vi "arduino_LM35.vi"() -> ()   [LabVIEW 2018]
uses:
  <vilib>/MakerHub/LINX/Public/Peripherals/Analog/Analog Read 1 Chan.vi
  <vilib>/MakerHub/LINX/Public/Peripherals/Analog/Analog Read N Chans.vi
  <vilib>/MakerHub/LINX/Private/Local IO/LinxAnalogRead.vi
  <vilib>/MakerHub/LINX/Public/Utilities/Check Channel.vi
  <vilib>/MakerHub/LINX/Private/Utilties/Generate Error.vi
  <vilib>/MakerHub/LINX/LMH-LINX.lvlib
panel:
  out "Sıcaklık":dbl
  in  "stop":bool
  out "Sıcaklık Grafiği":dbl(graph)
  out "Sıcaklık":dbl(slide) scale=0.0..100.0
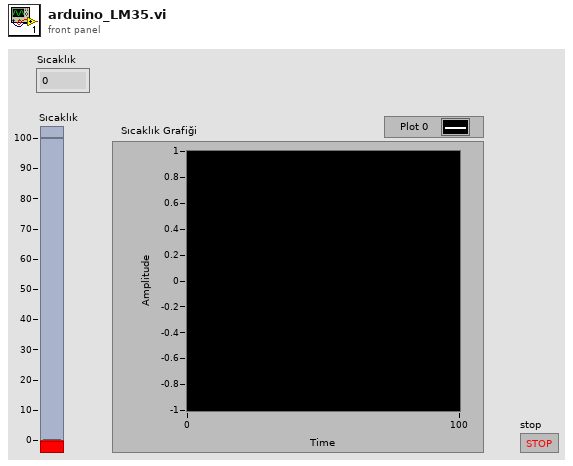
[diagram p1: front panel]
types:
  T1 = typedef "LMH-LINX.lvlib/LINX Ref.ctl" = cluster{"IO":T2, "Interface":T3, "LINX Device Config":T4}
  T2 = typedef "LMH-LINX.lvlib/Platform.ctl" = enum16{"Remote", "Local"}
  T3 = typedef "LMH-LINX.lvlib/Interface.ctl" = enum16{"Serial", "TCP"}
  T4 = typedef "LMH-LINX.lvlib/Device.lvlib/LINX Device Config.ctl" = cluster{"Interface":T3, "COM Port":refnum<visa-resource-name>, "TCP Configuration":T5, "Device Family":u8, "Device ID":u8, "Device Name":string, "TCP Ref":refnum<k5>, "Channels":T6}
  T5 = typedef "LMH-LINX.lvlib/Device.lvlib/TCP Config.ctl" = cluster{"IP Address":string, "Port":u16}
  T6 = typedef "LMH-LINX.lvlib/Channels.ctl" = cluster{"DI":u8[], "DO":u8[], "AI":u8[], "AO":u8[], "PWM":u8[], "QE":u8[], "UART":u8[], "I2C 2":u8[], "SPI":u8[], "CAN":u8[], "Servo":u8[], "AI Ref (V)":dbl, "AI Resolution (Bits)":u8, "AO Ref (V)":dbl, "AO Resolution (Bits)":u8}
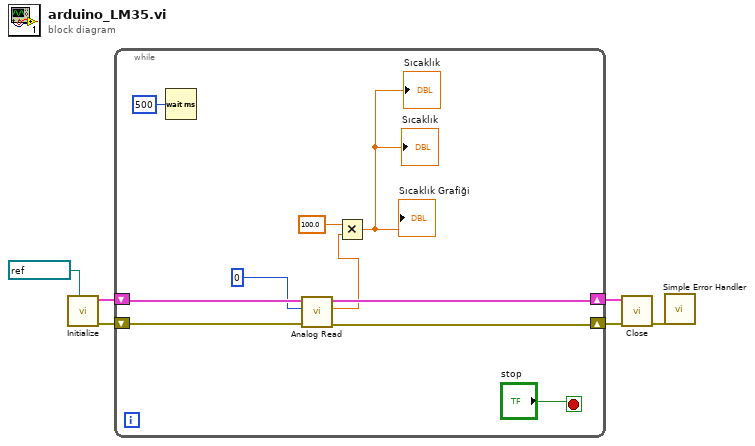
[diagram p0: block diagram]
diagram:
  n1 = call <vilib>:"Initialize.vi"("Serial Port"=refnum<visa-resource-name> "COM8") -> ("Error Out"=w6:errorcluster, "LINX Resource"=w4:T1)  [unwired: 8 in, 1 out]
  n2 = while {
    shift-right: [w15] -> w5
    shift-left: w6 -> [w16]
    shift-right: [w13] -> w3
    shift-left: w4 -> [w14]
    stop <- "stop" stop-if-true
    n3 = Wait (ms)(milliseconds to wait=u32 500) -> ()  [unwired: 1 out]
    n4 = call-poly <vilib>:"Analog Read.vi"("Error In"=w16, "Analog Channel"=u8 0, "LINX Resource"=w14) -> ("Error Out"=w15:errorcluster, "Voltage"=w8:dbl, "LINX Resource"=w13:T1)  [unwired: 5 in, 1 out]
    n5 = Multiply(x=100.0, y=w8) -> (x*y=→"Sıcaklık" →"Sıcaklık Grafiği" →"Sıcaklık":dbl)
  }
  n6 = call <vilib>:"Close.vi"("Error In"=w5, "LINX Resource"=w3) -> ("Error Out"=w1:errorcluster)  [unwired: 9 in]
  n7 = call <vilib>:"Simple Error Handler.vi"("error in (no error)"=w1) -> ()  [unwired: 4 in, 5 out]
